vi "Contol de autonomo global.vi"() -> ()   [LabVIEW 2014]
panel:
  in  "Reach the zone":bool
  in  "Ready to moonwalk":bool
  in  "Kissed the wall and i like it":bool
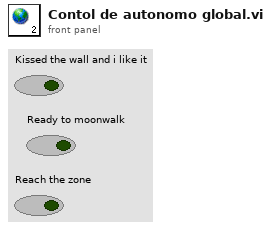
[diagram p1: front panel]
diagram:
